vi "struct_ref_dp_sat_dT_T.vi"(8 "Error (Input)":errorcluster, 10 "Temperature in K (Input)":dbl, 11 "Reference working pair (Input)":i64) -> (0 "Error (Output)":errorcluster, 3 "Der. of saturation pressure wrt temperature in Pa/K (Output)":dbl)   [LabVIEW 2017]
doc: "ref_dp_sat_dT_T:\n * ----------------\n *\n * Calculates derivative of saturation pressure in Pa/K wrt to temperature\n * depending on equilibrium temperature T in K.\n *\n * Parameters:\n * -----------\n * double T_K:\n * Equilibrium temperature in K.\n * struct *WorkingPair:\n * Pointer of WorkingPair-struct.\n *\n * Returns:\n * --------\n * double:\n * Derivative of saturation pressure wrt temperature in Pa/K.\n *\n * History:\n * --------\n *07/13/2021, by Jannik Driesel (supervised by Mirko Engelpracht)\n * First implementation."
uses:
  data/win32bit/libsorpPropLib.dll
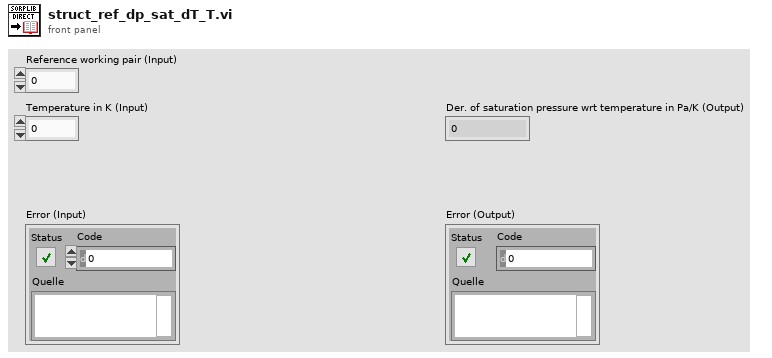
[diagram p1: front panel]
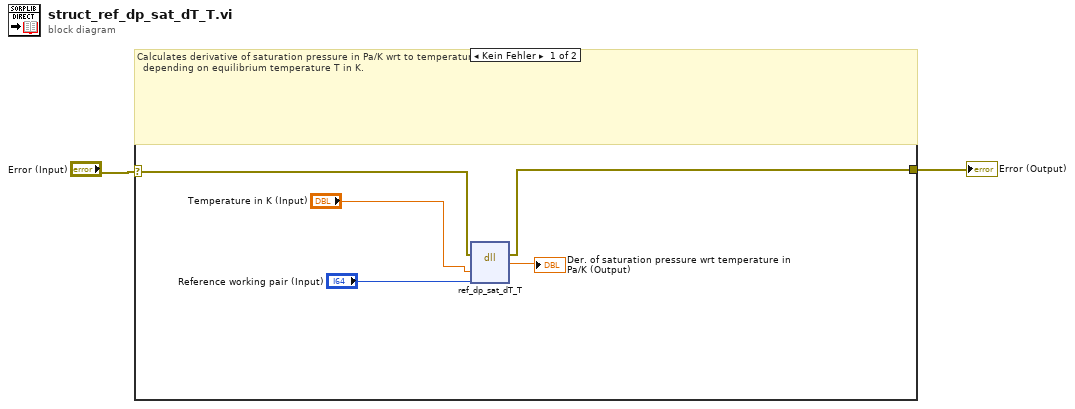
[diagram p0: block diagram]
diagram:
  n1 = case shown="Kein Fehler" "Error (Input)" {
    selector: "Error (Input)" -> [w7 w8]
    tunnel: [w6 w8] -> w2
    frame No Error {
      # "Calculates derivative of saturation pressure in Pa/K wrt to temperature\n  depending on equilibrium temperature T in K."
      n2 = dll-call lib="D:/Driesel/SorpLibLocal/LabVIEW_wrapper/data/win32bit/libsorpPropLib.dll" fn="ref_dp_sat_dT_T"(error in=w7, "T_K"="Temperature in K (Input)", "workingPair"="Reference working pair (Input)") -> (error out=w6:errorcluster, "dp_sat_dT"=→"Der. of saturation pressure wrt temperature in Pa/K (Output)":dbl)  [unwired: 4 in, 1 out]
    }
    frame Error {
      # "Error - No calculations"
    }
  }
  "Error (Output)" <- w2
